vi "Write configuration.vi"(8 "error in (no error)":errorcluster, 11 "ImageStack in":refnum<class "Invivo_ImageStack.lvclass">) -> (0 "error out":errorcluster, 3 "ImageStack out":refnum<class "Invivo_ImageStack.lvclass">)   [LabVIEW 2012, in "Invivo_ImageStack.lvclass"]
doc: "Writes the configuration cluster into the configuration file. Configuration file is XML-based. It's name is <component ID>.xml"
uses:
  Invivo_ImageStack.lvclass
  <vilib>/Distrio/Murmex/Murmex/Murmex.lvclass
  Invivo_ImageStack.lvclass/Invivo_ImageStack.ctl
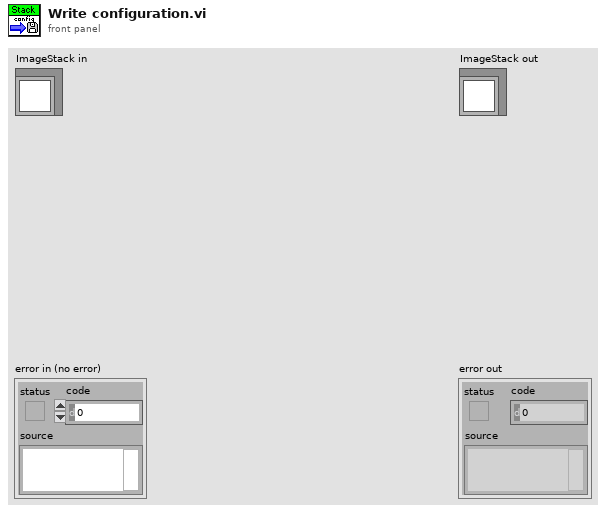
[diagram p1: front panel]
types:
  T1 = typedef "ImageStack.lvclass/configuration_cluster.ctl" = cluster{"Camera component name":string, "Stages component name":string, "AOTF component name":string}
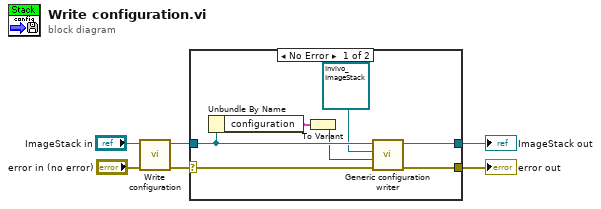
[diagram p0: block diagram]
diagram:
  n1 = call-parent "Write configuration.vi"("error in (no error)"="error in (no error)", "Murmex in"="ImageStack in") -> ("error out"=w4:errorcluster, "Murmex out"=w1:refnum<class "Invivo_ImageStack.lvclass">)  [unwired: 8 in]
  n2 = case shown="No Error" w4 {
    selector: w4 -> [w13 w15]
    tunnel: [w7 w15] -> w3
    tunnel: [w8 w14] -> w2
    tunnel: w1 -> [w12 w14]
    frame No Error {
      n3 = Unbundle By Name(w12) -> ("configuration"=w11:T1)
      n4 = To Variant(anything=w11) -> (Variant=w10:variant)
      n5 = call <vilib>:"Generic configuration writer.vi"("error in (no error)"=w13, "configuration"=w10, "inheritance level"=refnum<class "Invivo_ImageStack.lvclass"> refnum ("ImageStack"), "MurmexBase in"=w12) -> ("error out"=w7:errorcluster, "MurmexBase out"=w8:refnum<class "Invivo_ImageStack.lvclass">)  [unwired: 6 in]
    }
    frame Error {
    }
  }
  "error out" <- w3
  "ImageStack out" <- w2
